vi "Main LIEF Listbox.vi"() -> ()   [LabVIEW 2016]
uses:
  LIEF Listbox Handler/Listbox Handler.lvclass
  C:/Program Files (x86)/National Instruments/LabVIEW 2016/vi.lib/LIEF/Image Editor Handler/Image Editor Handler.lvclass
  LIEF Listbox Handler/Listbox Handler.lvclass/Listbox Handler.ctl
  <vilib>/LIEF/Forms/Shape/Shape.lvclass/Shape.ctl
  <vilib>/LIEF/Forms/Layered Shape/Layered Shape.lvclass/Layered Shape.ctl
  <vilib>/LIEF/Forms/Shape/Write Color.vi
  <vilib>/LIEF/Forms/Shape/Write Movable.vi
  <vilib>/LIEF/Forms/Layered Shape/Write Overlays.vi
  LIEF Listbox Handler/Write SelectionChanged Event.vi
  LIEF Listbox Handler/Write Pixel Step.vi
  <vilib>/LIEF/Forms/Text/Text.lvclass
  C:/Program Files (x86)/National Instruments/LabVIEW 2016/vi.lib/LIEF/Forms/Shape/Shape.lvclass
  <vilib>/LIEF/Forms/Rectangle/Rectangle.lvclass
  C:/Program Files (x86)/National Instruments/LabVIEW 2016/vi.lib/LIEF/Forms/Layered Shape/Layered Shape.lvclass
  <vilib>/LIEF/Image Editor Handler/Image Editor Handler.lvclass
  <vilib>/LIEF/Forms/Shape/Shape.lvclass
  <vilib>/LIEF/Forms/Grid/Grid.lvclass
panel:
  out "Selection":i32
  out "Array":string[](array[string])
  in  "2D Picture":picture
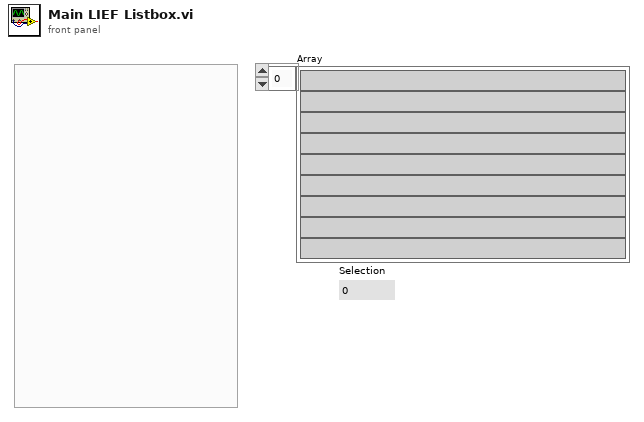
[diagram p1: front panel]
types:
  T1 = typedef "LVBoundsTypeDef.ctl" = cluster{"Width":u32, "Height":u32}
  T2 = enum16{"Left", "Top", "Right", "Bottom", "Centered"}
  T3 = typedef "eventvkey.ctl" = enum16{"ASCII", "Enter", "Return", "Shift", "Ctrl", "Alt", "Cmd", "Opt", "Caps", "NumLock", "Clear", "Break", "Up", "Down", "Left", "Right", "Insert", "Delete", "Home", "End", "PageUp", "PageDown", "Escape", "Help", "Pause", "ScrollLock", "F1", "F2", "F3", "F4", "F5", "F6", "F7", "F8", "F9", "F10", "F11", "F12", "F13", "F14", "F15", "F16", "F17", "F18", "F19", "F20", "F21", "F22", "F23", "F24", "Play", "VolumeUp", "VolumeDown", "Mute", "Two Byte Char"}
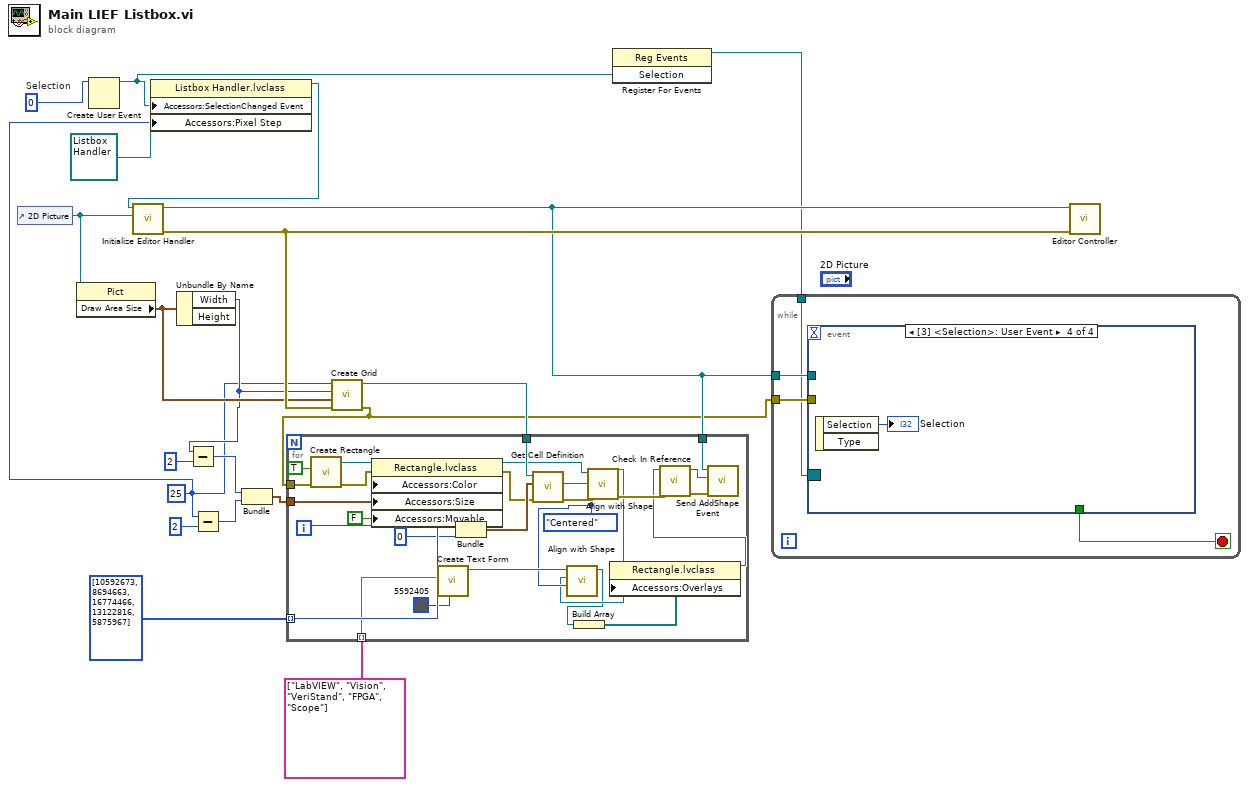
[diagram p0: block diagram]
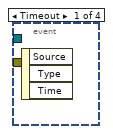
[diagram p2: hidden frame]
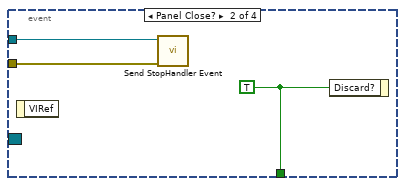
[diagram p3: hidden frame]
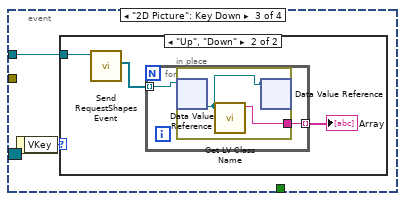
[diagram p4: hidden frame]
diagram:
  w6 = 0  # Selection
  w4 = u32 25 ("y")
  n1 = control-ref of="2D Picture"() -> (w20:refnum<vi>)
  n2 = property class="Pict"(reference=w20) -> ("Draw Area Size"=w17:T1)  [unwired: 1 in, 2 out]
  n3 = Create User Event(user event datatype=w6) -> (user event=w2:refnum<user-event>)  [unwired: 1 in, 1 out]
  n4 = property class="Listbox Handler.lvclass"(reference=refnum<class "Listbox Handler.lvclass"> refnum ("Listbox Handler.lvclass"), "Accessors:SelectionChanged Event"=w2, "Accessors:Pixel Step"=w4) -> (reference out=w3:refnum<class "Listbox Handler.lvclass">)  [unwired: 1 in, 1 out]
  n5 = call <vilib>:"Initialize Editor Handler.vi"("PictureRef"=w20, "Editor Handler in"=w3) -> ("error out"=w19:errorcluster, "Editor Handler out"=w18:refnum<class "Listbox Handler.lvclass">)  [unwired: 8 in]
  n6 = Unbundle By Name(w17) -> ("Width"=w9:u32)  [unwired: 1 out]
  n7 = Subtract(x=w9, y=u32 2) -> (x-y=w8:u32)
  n8 = Subtract(x=w4, y=u32 2) -> (x-y=w12:u32)
  n9 = Bundle(w8, w12) -> (w15:cluster{u32, u32})  [unwired: 1 in]
  n10 = call <vilib>:"Create Grid.vi"("error in (no error)"=w19, "Draw Area"=w17, "Horizontal Step"=w9, "Vertical Step"=w4) -> ("error out"=w11:errorcluster, "Grid Reference"=w14:refnum<data-value>)  [unwired: 6 in]
  n11 = for {
    tunnel: u32[] [10592673, 8694663, 16774466, 13122816, 5875967] ("Color") -> [w45] mode=indexing
    tunnel: w15 -> [w44]
    tunnel: w14 -> [w43]
    tunnel: w11 -> [w37]
    tunnel: w18 -> [w30]
    tunnel: string[] ["LabVIEW", "Vision", "VeriStand", "FPGA", "Scope"] ("Text") -> [w27] mode=indexing
    i -> [w42]
    w25 = T2."Centered" ("Alignment")
    n12 = call <vilib>:"Create Rectangle.vi"("error in (no error)"=w37, "Filled"=TRUE) -> ("error out"=w36:errorcluster, "Rectangle out"=w46:refnum<class "Rectangle.lvclass">)  [unwired: 8 in]
    n13 = property class="Rectangle.lvclass"(reference=w46, error in=w36, "Accessors:Color"=w45, "Accessors:Size"=w44, "Accessors:Movable"=FALSE ("Movable")) -> (reference out=w38:refnum<class "Rectangle.lvclass">, error out=w35:errorcluster)
    n14 = call <vilib>:"Create Text Form.vi"("Color"=u32 5592405, "Text"=w27) -> ("New Text"=w26:refnum<class "Text.lvclass">)  [unwired: 8 in, 1 out]
    n15 = Bundle(w42, "y"=u32 0) -> (w40:cluster{i32, "y":u32})  [unwired: 1 in]
    n16 = call <vilib>:"Get Cell Definition.vi"("error in (no error)"=w35, "Indexes"=w40, "Shape Reference"=w43) -> ("error out"=w34:errorcluster, "Cell"=w39:refnum<class "Shape.lvclass">)  [unwired: 6 in, 1 out]
    n17 = call <vilib>:"Align with Shape.vi"("error in (no error)"=w34, "Alignment"=w25, "Reference Shape"=w39, "Shape in"=w38) -> ("error out"=w33:errorcluster, "Shape out"=w24:refnum<class "Rectangle.lvclass">)  [unwired: 6 in]
    n18 = call <vilib>:"Align with Shape.vi"("Alignment"=w25, "Reference Shape"=w24, "Shape in"=w26) -> ("Shape out"=w23:refnum<class "Text.lvclass">)  [unwired: 7 in, 1 out]
    n19 = Build Array(w23) -> (w22:refnum<class "Text.lvclass">[])
    n20 = property class="Rectangle.lvclass"(reference=w24, "Accessors:Overlays"=w22) -> (reference out=w21:refnum<class "Rectangle.lvclass">)  [unwired: 1 in, 1 out]
    n21 = call <vilib>:"Check In Reference.vi"("error in (no error)"=w33, "Shape in"=w21) -> ("error out"=w32:errorcluster, "Shape Reference"=w31:refnum<data-value>)  [unwired: 8 in]
    n22 = call <vilib>:"Send AddShape Event.vi"("error in (no error)"=w32, "New Shape Reference"=w31, "Editor Handler in"=w30) -> ()  [unwired: 7 in, 2 out]
  }
  n23 = register-events(w2) -> (reference out=w1:refnum<event-registration>)  [unwired: 2 in, 1 out]
  n24 = while {
    tunnel: w18 -> [w50]
    tunnel: w11 -> [w49]
    tunnel: w1 -> [w48]
    stop <- w51 stop-if-true
    n25 = event shown="[3] <Selection>: User Event" {
      selector: w48 -> [_ _ _ _]
      dyn-events: _ -> [_ _ _ _]
      timeout: _ -> [_ _ _ _]
      tunnel: [_ w54 _ _] -> w51
      tunnel: w50 -> [_ w53 w55 _]
      tunnel: w49 -> [_ w52 _ _]
      event Timeout {
        n26 = event-data() -> ()  [unwired: 1 in, 3 out]
      }
      event Panel Close? {
        w54 = TRUE ("Discard?")
        n27 = event-data() -> ()  [unwired: 1 in, 1 out]
        n28 = call <vilib>:"Send StopHandler Event.vi"("error in (no error)"=w52, "Editor Handler in"=w53) -> ()  [unwired: 8 in, 2 out]
        n29 = event-data("Discard?"=w54) -> ()  [unwired: 1 in, 1 out]
      }
      event "2D Picture": Key Down {
        n30 = event-data() -> ("VKey"=w56:T3)  [unwired: 1 in]
        n31 = case shown="\"Up\", \"Down\"" w56 {
          tunnel: w55 -> [_ w59]
          frame "ASCII", Default {
          }
          frame "Up", "Down" {
            n32 = call <vilib>:"Send RequestShapes Event.vi"("Editor Handler in"=w59) -> ("Shapes"=w58:refnum<data-value>[])  [unwired: 8 in, 2 out]
            n33 = for {
              tunnel: w58 -> [w61] mode=indexing
              tunnel: [w60] -> w57 mode=indexing
              n34 = in-place {
                in-place-border: [w62] -> w60
                n35 = in-place-dvr #1(w61) -> (w63:refnum<class "Shape.lvclass">)  [unwired: 1 out]
                n36 = call <vilib>:"Get LV Class Name.vi"("object"=w63) -> ("class name"=w62:string)  [unwired: 9 in, 1 out]
                n37 = in-place-dvr #1(w63) -> ()  [unwired: 2 out]
              }
            }
            "Array" <- w57
          }
        }
      }
      event User Event {
        n38 = event-data() -> ("Selection"=→"Selection":i32)  [unwired: 1 in, 1 out]
      }
    }
  }
  n39 = call <vilib>:"Editor Controller.vi"("error in (no error)"=w19, "Editor Handler in"=w18) -> ()  [unwired: 8 in, 2 out]
